vi "9235_UI.vi"(8 "error in (no error)":errorcluster, 11 "Node Ptr":T3 format="%.0x") -> (0 "error out":errorcluster)   [LabVIEW 2020, in "Modules.lvlib" / "9235.lvclass"]
uses:
  9235.lvclass
  <vilib>/NI VeriStand/Custom Device API/Custom Device Item Ref.ctl
  RSI Module/SubPanel Command.ctl
  AI Settings.ctl
  Data rate.ctl
  C:/Users/nitest/Desktop/Git 2020/niveristand-scan-engine-module-libraries/Source/RSI Module/RSI Module.lvclass
  9235.lvclass/9235.ctl
  RSI Module/RSI Module.lvclass
  <vilib>/NI VeriStand/Custom Device API/Custom Device API.lvlib
panel:
  in  "ADC sampling rate":T1 items=["10.000 kS/s", "8.333 kS/s", "7.143 kS/s", "6.250 kS/s", "5.556 kS/s", "5.000 kS/s", "4.545 kS/s", "4.167 kS/s", "3.846 kS/s", "3.571 kS/s", "3.333 kS/s", "3.125 kS/s", "2.941 kS/s", "2.778 kS/s", "2.632 kS/s", "2.500 kS/s", "2.381 kS/s", "2.273 kS/s", "2.174 kS/s", "2.083 kS/s", "2.000 kS/s", "1.923 kS/s", "1.852 kS/s", "1.786 kS/s", "1.724 kS/s", "1.667 kS/s", "1.613 kS/s", "1.563 kS/s", "1.515 kS/s", "1.471 kS/s", "1.429 kS/s", "1.389 kS/s", "1.351 kS/s", "1.316 kS/s", "1.282 kS/s", "1.250 kS/s", "1.220 kS/s", "1.190 kS/s", "1.163 kS/s", "1.136 kS/s", "1.136 kS/s", "1.111 kS/s", "1.087 kS/s", "1.064 kS/s", "1.042 kS/s", "1.020 kS/s", "1.000 kS/s", "980 S/s", "962 S/s", "943 S/s", "926 S/s", "909 S/s", "893 S/s", "877 S/s", "862 S/s", "847 S/s", "833 S/s", "820 S/s", "806 S/s", "794 S/s"]
  in  "Dynamic shunt?":bool
  in  "AI Settings":T2
  in  "SubPanel Event":refnum<user-event>
  in  "Header":cluster{"Section Name":string}={"Section Name"="NI 9205 Settings"}
  # "Shunt Calibration\n      Enabled"
  # "AI 0"
  # "AI 1"
  # "AI 2"
  # "AI 3"
  # "AI 4"
  # "AI 5"
  # "AI 6"
  # "AI 7"
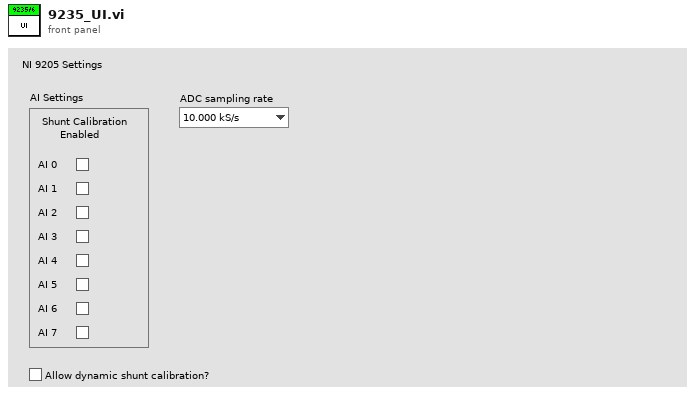
[diagram p1: front panel]
types:
  T1 = typedef "Modules.lvlib/9235.lvclass/Data rate.ctl" = u32
  T2 = typedef "Modules.lvlib/9235.lvclass/AI Settings.ctl" = cluster{"AI0 Shunt":bool, "AI1 Shunt":bool, "AI2 Shunt":bool, "AI3 Shunt":bool, "AI4 Shunt":bool, "AI5 Shunt":bool, "AI6 Shunt":bool, "AI7 Shunt":bool}
  T3 = typedef "Custom Device API.lvlib/Custom Device Item Ref.ctl" = u64
  T4 = typedef "Modules.lvlib/RSI Module.lvclass/Module Models.ctl" = enum16{"Empty", "NI 9201", "NI 9203", "NI 9205", "NI 9206", "NI 9207", "NI 9208", "NI 9209", "NI 9210", "NI 9211", "NI 9212", "NI 9213", "NI 9214", "NI 9215", "NI 9216", "NI 9217", "NI 9219", "NI 9220", "NI 9221", "NI 9222", "NI 9223", "NI 9224", "NI 9225", "NI 9226", "NI 9227", "NI 9228", "NI 9229", "NI 9233", "NI 9234", "NI 9235", "NI 9236", "NI 9237", "NI 9239", "NI 9242", "NI 9244", "NI 9253", "NI 9263", "NI 9264", "NI 9265", "NI 9266", "NI 9269", "NI 9344", "NI 9350", "NI 9375", "NI 9401", "NI 9402", "NI 9403", "NI 9411", "NI 9421", "NI 9422", "NI 9423", "NI 9425", "NI 9426", "NI 9435", "NI 9436", "NI 9437", "NI 9472", "NI 9474", "NI 9475", "NI 9476", "NI 9477", "NI 9478", "NI 9481", "NI 9482", "NI 9485"}
  T5 = typedef "Modules.lvlib/RSI Module.lvclass/SubPanel Command.ctl" = enum16{"Stop"}
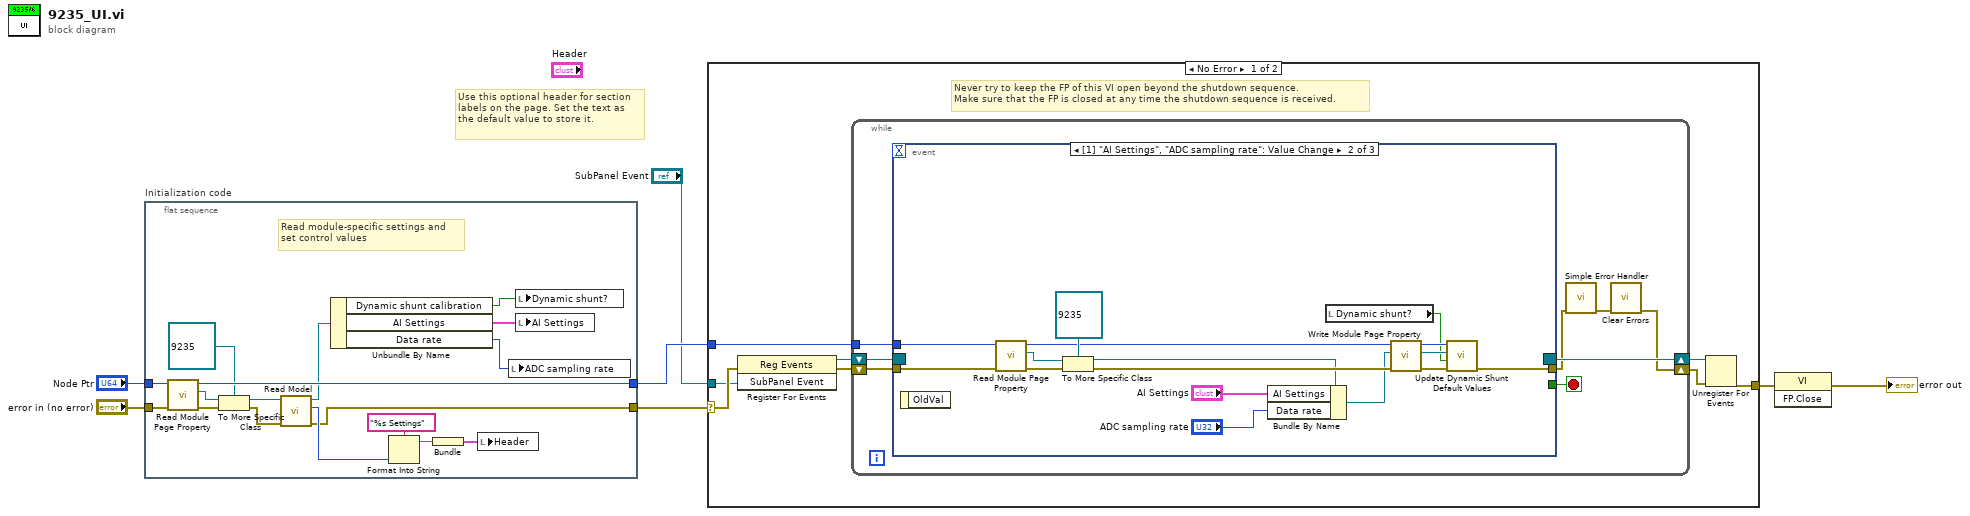
[diagram p0: block diagram]
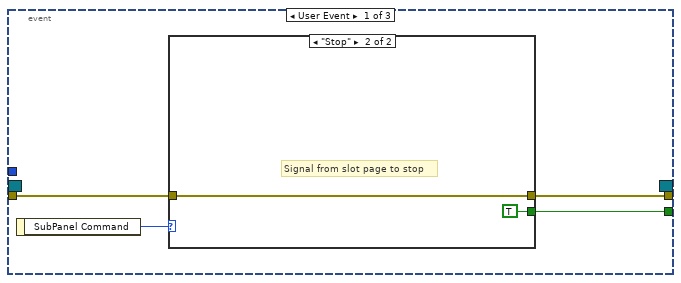
[diagram p2: hidden frame]
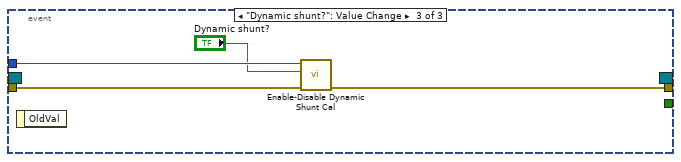
[diagram p4: hidden frame]
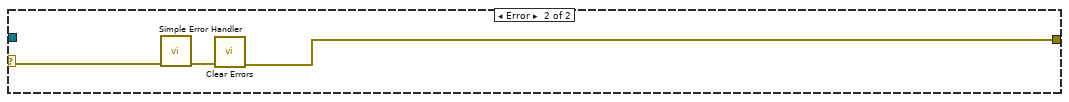
[diagram p5: hidden frame]
diagram:
  # "Use this optional header for section labels on the page. Set the text as the default value to store it."
  n1 = flat-sequence "Initialization code" {
    tunnel: "error in (no error)" -> [w23]
    tunnel: "Node Ptr" -> [w24]
    tunnel: [w11] -> w1
    tunnel: [w22] -> w4
    frame #0 {
      # "Read module-specific settings and\nset control values"
      n2 = call "Read Module Page Property.vi"("error in (no error)"=w23, "Node Ptr In"=w24) -> ("error out"=w21:errorcluster, "RSI Module"=w19:refnum<class "RSI Module.lvclass">, "Node Ptr Out"=w22:T3)  [unwired: 7 in]
      n3 = To More Specific Class(target class=refnum<class "9235.lvclass"> refnum ("9205 in"), reference=w19, error in=w21) -> (specific class reference=w18:refnum<class "9235.lvclass">, error out=w17:errorcluster)
      n4 = call "Read Model.vi"("error in (no error)"=w17, "RSI Module in"=w18) -> ("error out"=w11:errorcluster, "Model"=w15:T4, "RSI Module out"=w12:refnum<class "9235.lvclass">)  [unwired: 7 in]
      n5 = Unbundle By Name(w12) -> ("Dynamic shunt calibration"=w9:bool, "AI Settings"=w10:T2, "Data rate"=w8:T1)
      n6 = Format Into String(format string="%s Settings", w15) -> (resulting string=w13:string)  [unwired: 2 in, 1 out]
      n7 = Bundle(w13) -> (w16:cluster{string})  [unwired: 1 in]
      n8 = local write "Header"(w16) -> ()
      n9 = local write "ADC sampling rate"(w8) -> ()
      n10 = local write "Dynamic shunt?"(w9) -> ()
      n11 = local write "AI Settings"(w10) -> ()
    }
  }
  n12 = case shown="No Error" w1 {
    selector: w1 -> [w26 w70]
    tunnel: [w30 w68] -> w7
    tunnel: w4 -> [w27 _]
    tunnel: "SubPanel Event" -> [w25 _]
    frame No Error {
      # "Never try to keep the FP of this VI open beyond the shutdown sequence.\nMake sure that the FP is closed at any time the shutdown sequence is received."
      n13 = register-events(error in=w26, w25) -> (reference out=w28:refnum<event-registration>, error out=w29:errorcluster)  [unwired: 1 in]
      n14 = while {
        tunnel: w27 -> [w36]
        shift-right: [w33] -> w31
        shift-left: w29 -> [w39]
        shift-right: [w40] -> w32
        shift-left: w28 -> [w38]
        stop <- w37 stop-if-true
        n15 = event shown="[1] \"AI Settings\", \"ADC sampling rate\": Value Change" {
          selector: w38 -> [_ _ _]
          dyn-events: [_ _ _] -> w40
          timeout: _ -> [_ _ _]
          tunnel: w39 -> [w43 w58 w67]
          tunnel: [w42 _ _] -> w37
          tunnel: [w41 w52 w64] -> w35
          tunnel: w36 -> [_ w59 w66]
          event User Event {
            n16 = event-data() -> ("SubPanel Command"=w44:T5)  [unwired: 1 out]
            n17 = case shown="\"Stop\"" w44 {
              tunnel: w43 -> [w45 w46]
              tunnel: [w45 w46] -> w41
              tunnel: [_ TRUE] -> w42
              frame Default {
              }
              frame "Stop" {
                # "Signal from slot page to stop"
              }
            }
          }
          event Value Change {
            n18 = event-data() -> ()  [unwired: 2 out]
            n19 = call "Read Module Page Property.vi"("error in (no error)"=w58, "Node Ptr In"=w59) -> ("error out"=w61:errorcluster, "RSI Module"=w62:refnum<class "RSI Module.lvclass">, "Node Ptr Out"=w60:T3)  [unwired: 7 in]
            n20 = To More Specific Class(target class=refnum<class "9235.lvclass"> refnum ("9205 in"), reference=w62, error in=w61) -> (specific class reference=w56:refnum<class "9235.lvclass">, error out=w57:errorcluster)
            n21 = Bundle By Name(cluster=w56, "AI Settings"="AI Settings", "Data rate"="ADC sampling rate") -> (w54:refnum<class "9235.lvclass">)
            n22 = local read "Dynamic shunt?"() -> (w49:bool)
            n23 = call "Write Module Page Property.vi"("error in (no error)"=w57, "RSI Module"=w54, "Node Ptr In"=w60) -> ("error out"=w53:errorcluster, "RSI Module out"=w51:refnum<class "9235.lvclass">, "Node Ptr Out"=w50:T3)  [unwired: 6 in]
            n24 = call "Update Dynamic Shunt Default Values.vi"("error in (no error)"=w53, "Dynamic shunt?"=w49, "9235 in"=w51, "Node Ptr in"=w50) -> ("error out"=w52:errorcluster)  [unwired: 5 in, 2 out]
          }
          event "Dynamic shunt?": Value Change {
            n25 = event-data() -> ()  [unwired: 2 out]
            n26 = call "Enable-Disable Dynamic Shunt Cal.vi"("error in"=w67, "Dynamic shunt?"="Dynamic shunt?", "Node Ptr in"=w66) -> ("error out"=w64:errorcluster)  [unwired: 7 in, 1 out]
          }
        }
        n27 = call <vilib>:"Simple Error Handler.vi"("error in (no error)"=w35) -> ("error out"=w34:errorcluster)  [unwired: 1 in, 7 out]
        n28 = call <vilib>:"Clear Errors.vi"("error in (no error)"=w34) -> ("error out"=w33:errorcluster)  [unwired: 1 in, 5 out]
      }
      n29 = Unregister For Events(event registration refnum=w32, error in=w31) -> (error out=w30:errorcluster)
    }
    frame Error {
      n30 = call <vilib>:"Simple Error Handler.vi"("error in (no error)"=w70) -> ("error out"=w69:errorcluster)  [unwired: 1 in, 7 out]
      n31 = call <vilib>:"Clear Errors.vi"("error in (no error)"=w69) -> ("error out"=w68:errorcluster)  [unwired: 1 in, 5 out]
    }
  }
  n32 = invoke class="VI" method="FP.Close"(error in=w7) -> (error out=→"error out":errorcluster)  [unwired: 2 in, 2 out]
